vi "m_close.vi"(2 "error in (no error)":errorcluster, 3 "configuration file path":path) -> (0 "error out":errorcluster, 1 "configuration file path copy":path)   [LabVIEW 2017]
doc: "Save Cornerstone parameters to configuration (INI) file."
uses:
  m_globals.vi
  <vilib>/Utility/config.llb/NI_LVConfig.lvlib
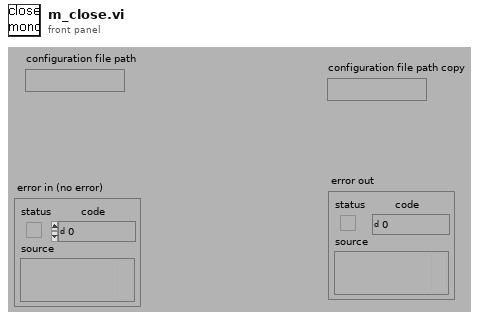
[diagram p1: front panel]
types:
  T1 = typedef "NI_LVConfig.lvlib/Config Data RefNum.ctl" = refnum<k1>
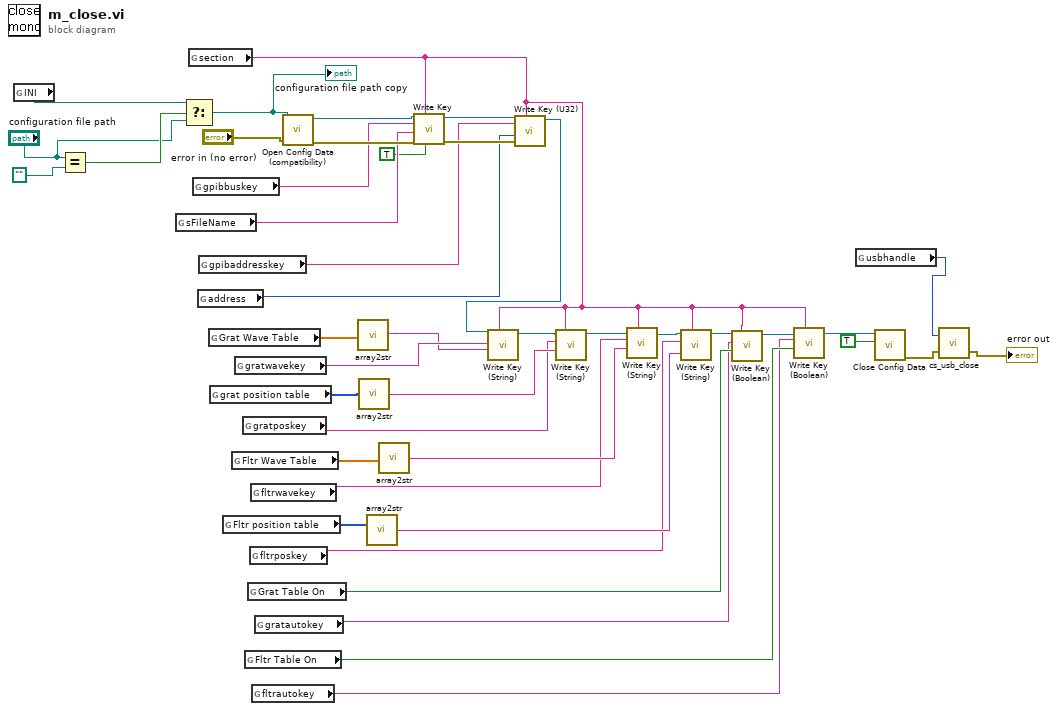
[diagram p0: block diagram]
diagram:
  n1 = global read "m_globals.vi" "INI"() -> (w6:path)
  n2 = Equal?(x="configuration file path", y=path "") -> (x = y?=w8:bool)
  n3 = global read "m_globals.vi" "sFileName"() -> (w34:string)
  n4 = Select(t=w6, s=w8, f="configuration file path") -> (s? t:f=w5:path)
  "configuration file path copy" <- w5
  n5 = global read "m_globals.vi" "section"() -> (w23:string)
  n6 = global read "m_globals.vi" "gpibbuskey"() -> (w37:string)
  n7 = global read "m_globals.vi" "address"() -> (w35:i16)
  n8 = global read "m_globals.vi" "gpibaddresskey"() -> (w36:string)
  n9 = global read "m_globals.vi" "Grat Wave Table"() -> (w33:dbl[])
  n10 = global read "m_globals.vi" "grat position table"() -> (w32:u16[])
  n11 = global read "m_globals.vi" "Fltr position table"() -> (w30:u16[])
  n12 = global read "m_globals.vi" "Fltr Wave Table"() -> (w31:dbl[])
  n13 = global read "m_globals.vi" "gratwavekey"() -> (w22:string)
  n14 = global read "m_globals.vi" "gratposkey"() -> (w19:string)
  n15 = global read "m_globals.vi" "Fltr Table On"() -> (w12:bool)
  n16 = global read "m_globals.vi" "Grat Table On"() -> (w14:bool)
  n17 = global read "m_globals.vi" "fltrposkey"() -> (w15:string)
  n18 = global read "m_globals.vi" "fltrwavekey"() -> (w17:string)
  n19 = global read "m_globals.vi" "fltrautokey"() -> (w11:string)
  n20 = global read "m_globals.vi" "gratautokey"() -> (w13:string)
  n21 = call <vilib>:"Open Config Data (compatibility).vi"("error in (no error)"="error in (no error)", "configuration file path"=w5) -> ("error out"=w41:errorcluster, "refnum"=w43:T1)  [unwired: 7 in, 1 out]
  n22 = call "array2str.vi"("array in"=w33) -> ("string out"=w21:string)
  n23 = call "array2str.vi"("array in"=w32) -> ("string out"=w20:string)
  n24 = call "array2str.vi"("array in"=w30) -> ("string out"=w16:string)
  n25 = call "array2str.vi"("array in"=w31) -> ("string out"=w18:string)
  n26 = call-poly <vilib>:"Write Key.vi"("write raw string? (F)"=TRUE, "section"=w23, "error in (no error)"=w41, "value"=w34, "key"=w37, "refnum"=w43) -> ("error out"=w40:errorcluster, "refnum out"=w39:T1)  [unwired: 3 in, 1 out]
  n27 = call <vilib>:"Write Key (U32).vi"("section"=w23, "error in (no error)"=w40, "value"=w35, "key"=w36, "refnum"=w39) -> ("refnum out"=w29:T1)  [unwired: 4 in, 2 out]
  n28 = call <vilib>:"Write Key (String).vi"("section"=w23, "value"=w21, "key"=w22, "refnum"=w29) -> ("refnum out"=w28:T1)  [unwired: 5 in, 2 out]
  n29 = call <vilib>:"Write Key (String).vi"("section"=w23, "value"=w20, "key"=w19, "refnum"=w28) -> ("refnum out"=w27:T1)  [unwired: 5 in, 2 out]
  n30 = call <vilib>:"Write Key (String).vi"("section"=w23, "value"=w18, "key"=w17, "refnum"=w27) -> ("refnum out"=w26:T1)  [unwired: 5 in, 2 out]
  n31 = call <vilib>:"Write Key (String).vi"("section"=w23, "value"=w16, "key"=w15, "refnum"=w26) -> ("refnum out"=w25:T1)  [unwired: 5 in, 2 out]
  n32 = call <vilib>:"Write Key (Boolean).vi"("section"=w23, "value"=w14, "key"=w13, "refnum"=w25) -> ("refnum out"=w24:T1)  [unwired: 5 in, 2 out]
  n33 = call <vilib>:"Write Key (Boolean).vi"("section"=w23, "value"=w12, "key"=w11, "refnum"=w24) -> ("refnum out"=w10:T1)  [unwired: 5 in, 2 out]
  n34 = global read "m_globals.vi" "usbhandle"() -> (w2:i32)
  n35 = call <vilib>:"Close Config Data.vi"("write file if changed (T)"=TRUE ("write configuration file? (F)"), "refnum"=w10) -> ("error out"=w4:errorcluster)  [unwired: 8 in, 1 out]
  n36 = call "cs_usb_close.vi"("error in (no error)"=w4, "cs_usb handle"=w2) -> ("error out"=→"error out":errorcluster)  [unwired: 1 out]
